vi "MU Calibration Get Relative Nonius Track Adjustments.vi"(8 "error in (no error)":errorcluster, 11 "CalibrationAnalyzeResult":T2) -> (0 "error out (no error)":errorcluster, 3 "MU_Calibration_RelativeAnalogTrackAdjustments_Nonius":T1)   [LabVIEW 2017, in "MU_3SL_interface.lvlib"]
uses:
  MU_3SL_interface.lvlib
  handles/CalibrationAnalyzeResultHandle.ctl
  lib/MU_3SL_interface.dll
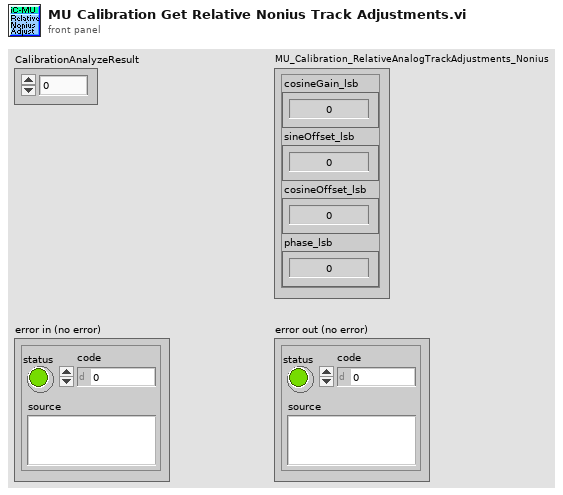
[diagram p1: front panel]
types:
  T1 = cluster{"cosineGain_lsb":dbl, "sineOffset_lsb":dbl, "cosineOffset_lsb":dbl, "phase_lsb":dbl}
  T2 = typedef "MU_3SL_interface.lvlib/CalibrationAnalyzeResultHandle.ctl" = u64
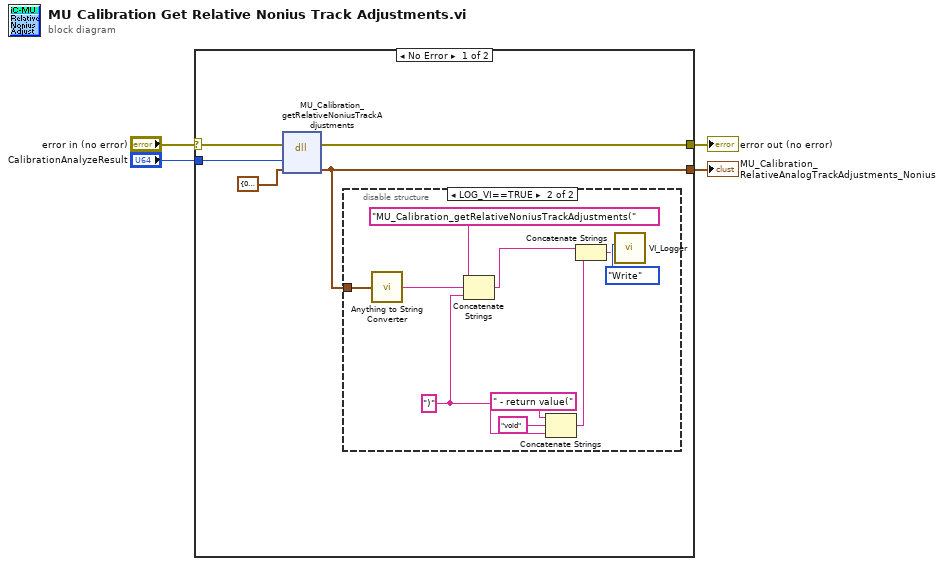
[diagram p0: block diagram]
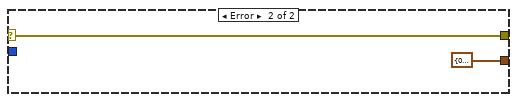
[diagram p3: hidden frame]
diagram:
  n1 = case shown="No Error" "error in (no error)" {
    selector: "error in (no error)" -> [w9 w21]
    tunnel: [w7 w21] -> w4
    tunnel: "CalibrationAnalyzeResult" -> [w8 _]
    tunnel: [w6 T1 {"cosineGain_lsb"=0.0, "sineOffset_lsb"=0.0, "cosineOffset_lsb"=0.0, "phase_lsb"=0.0} ("MU_Calibration_RelativeAnalogTrackAdjustments_Nonius")] -> w1
    frame No Error {
      n2 = dll-call lib="C:/Users/bes/AppData/Roaming/work/mu_9so/icsubmodules/soft_mu_3sl_master/lv_interface/lib/MU_3SL_interface**.*" fn="MU_Calibration_getRelativeNoniusTrackAdjustments"(error in=w9, "analyzeResult"=w8, "RelativeAnalogTrackAdjustments_Nonius"=T1 {"cosineGain_lsb"=0.0, "sineOffset_lsb"=0.0, "cosineOffset_lsb"=0.0, "phase_lsb"=0.0} ("MU_Calibration_RelativeAnalogTrackAdjustments_Nonius")) -> (error out=w7:errorcluster, "RelativeAnalogTrackAdjustments_Nonius"=w6:T1)  [unwired: 4 in, 1 out]
      n3 = disable-structure shown="LOG_VI==TRUE" {
        disable-tunnel: w6 -> [_ w12]
        frame condition #0 {
        }
        frame condition #1 (active) {
          w14 = ")" ("string")
          n4 = call "Anything to String Converter.vi"("anything"=w12) -> ("String"=w11:string)
          n5 = Concatenate Strings("MU_Calibration_getRelativeNoniusTrackAdjustments(" ("Info in"), w11, w14) -> (w10:string)
          n6 = Concatenate Strings(" - return value(" ("string"), "void" ("string"), w14) -> (w17:string)
          n7 = Concatenate Strings(w10, w17) -> (w16:string)
          n8 = call "VI_Logger.vi"("Action (Read)"=enum16{"Write", "Read"}."Write", "Info in"=w16) -> ()  [unwired: 8 in, 2 out]
        }
      }
    }
    frame Error {
    }
  }
  "error out (no error)" <- w4
  "MU_Calibration_RelativeAnalogTrackAdjustments_Nonius" <- w1
